vi "points_to_semicolon_delimited_string.vi"(11 "Array":cluster{"X":dbl, "Y":dbl}[](array[cluster])) -> (3 "delimited string":string)   [LabVIEW 2019]
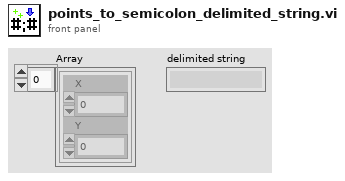
[diagram p1: front panel]
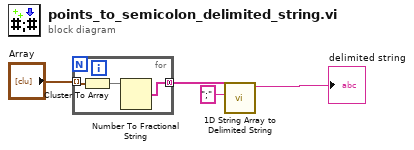
[diagram p0: block diagram]
diagram:
  n1 = for {
    tunnel: "Array" -> [w7] mode=indexing
    tunnel: [w5] -> w3 mode=concatenating
    n2 = Cluster To Array(cluster=w7) -> (array=w6:dbl[])
    n3 = Number To Fractional String(number=w6) -> (F-format string=w5:string[])  [unwired: 3 in]
  }
  n4 = call <vilib>:"1D String Array to Delimited String.vi"("delimiter"=";", "string array"=w3) -> ("delimited string"=→"delimited string":string)  [unwired: 9 in]
